vi "AD7609 config.vi"(4 "Timeout for software trig. mode (ms)":u32=15000, 5 "Device serial port":refnum<visa-resource-name>, 6 "Triggering mode":u8(ring) items=["Software", "Hardware, falling edge", "Hardware, rising edge"], 7 "N channels to read":u8(ring)=8 items=["1"=1, "2"=2, "3"=3, "4"=4, "5"=5, "6"=6, "7"=7, "8"=8], 8 "Input voltage range (V)":u8(ring)=1 items=["-5... +5 V", "-10... +10 V"], 9 "Oversampling ratio":u8(ring) items=["1", "2", "4", "8", "16", "32", "64"], 10 "Sampling rate (Hz)":sgl=1000.0, 11 "Number of samples":u32=1000) -> (0 "Config error out":errorcluster, 3 "Config read-back ok":bool=TRUE)   [LabVIEW 2016]
uses:
  <vilib>/Instr/_visa.llb/VISA Open Access Mode.ctl
  AD7609 global.vi
panel:
  out "Configuration read-back":string
  out "Configuration output":string
  # "56 kHz max. 8Ch\n80 kHz max. 1Ch"
  # "PN 25/11/2014, 17/08/2015, 23/08/2016, 03/09/2017"
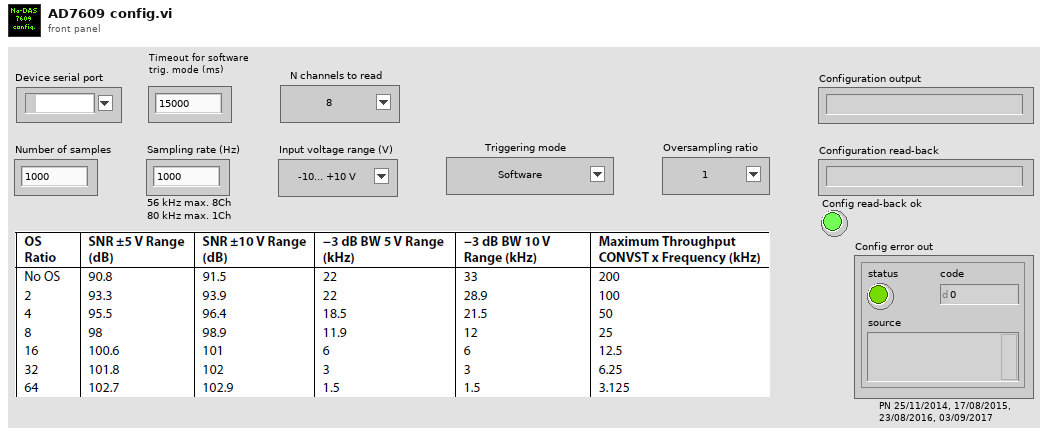
[diagram p1: front panel]
types:
  T1 = typedef "VISA Open Access Mode.ctl" = u32
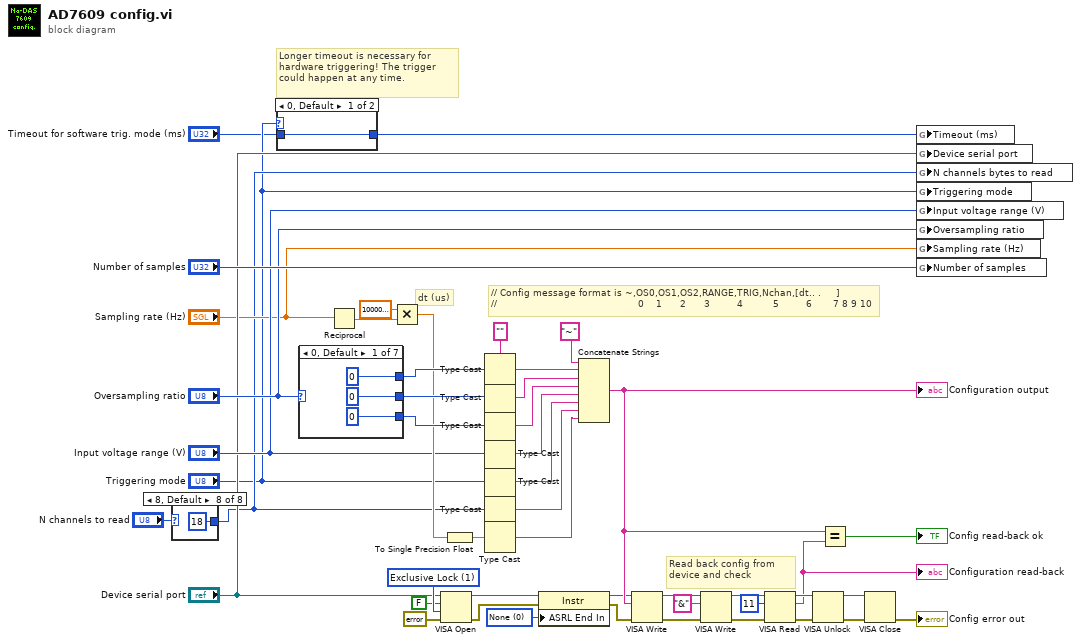
[diagram p0: block diagram]
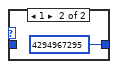
[diagram p2: hidden frame]
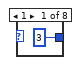
[diagram p3: hidden frame]
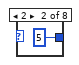
[diagram p4: hidden frame]
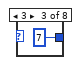
[diagram p5: hidden frame]
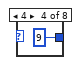
[diagram p6: hidden frame]
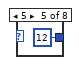
[diagram p7: hidden frame]
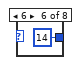
[diagram p8: hidden frame]
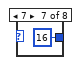
[diagram p9: hidden frame]
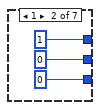
[diagram p10: hidden frame]
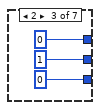
[diagram p11: hidden frame]
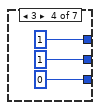
[diagram p12: hidden frame]
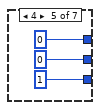
[diagram p13: hidden frame]
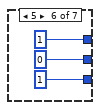
[diagram p14: hidden frame]
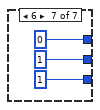
[diagram p15: hidden frame]
diagram:
  w8 = u16 0 items=["None", "Last Bit", "TermChar"] ("Serial Settings:End Mode for Reads")
  w36 = T1 1 items=["VISA Defaults"=0, "Exclusive Lock"=1, "Load Configured Settings"=4] ("Access Mode")
  w12 = ""
  # "Longer timeout is necessary for hardware triggering! The trigger could happen at any time."
  # "Read back config from device and check"
  # "// Config message format is ~,OS0,OS1,OS2,RANGE,TRIG,Nchan,[dt.. .     ]\n//                                               0    1      2      3         4          5         6       7 8 9 10"
  # "dt (us)"
  n1 = case shown="8, Default" "N channels to read" {
    tunnel: [u8 3 u8 5 u8 7 u8 9 u8 12 u8 14 u8 16 u8 18] -> w9
    frame 1 {
    }
    frame 2 {
    }
    frame 3 {
    }
    frame 4 {
    }
    frame 5 {
    }
    frame 6 {
    }
    frame 7 {
    }
    frame 8, Default {
    }
  }
  n2 = case shown="0, Default" "Triggering mode" {
    tunnel: [w57 u32 4294967295 ("Timeout (ms)")] -> w2
    tunnel: "Timeout for software trig. mode (ms)" -> [w57 _]
    frame 0, Default {
    }
    frame 1 {
    }
  }
  n3 = case shown="0, Default" "Oversampling ratio" {
    tunnel: [u8 0 u8 1 u8 0 u8 1 u8 0 u8 1 u8 0] -> w47
    tunnel: [u8 0 u8 0 u8 1 u8 1 u8 0 u8 0 u8 1] -> w46
    tunnel: [u8 0 u8 0 u8 0 u8 0 u8 1 u8 1 u8 1] -> w45
    frame 0, Default {
    }
    frame 1 {
    }
    frame 2 {
    }
    frame 3 {
    }
    frame 4 {
    }
    frame 5 {
    }
    frame 6 {
    }
  }
  n4 = Reciprocal(x="Sampling rate (Hz)") -> (1/x=w39:sgl)
  n5 = Multiply(x=sgl 1000000.0, y=w39) -> (x*y=w37:sgl)
  n6 = VISA Open(duplicate session (F)=FALSE, access mode=w36, error in (no error)=errorcluster {"status"=FALSE, "code"=0, "source"=""}, VISA resource name="Device serial port") -> (VISA resource name=w7:refnum<visa-resource-name>, error out=w4:errorcluster)  [unwired: 1 in]
  n7 = To Single Precision Float(number=w37) -> (single precision float=w25:sgl)
  n8 = Type Cast(type=w12, x=w47) -> (*(type *) &x=w44:string)
  n9 = Type Cast(type=w12, x=w46) -> (*(type *) &x=w43:string)
  n10 = Type Cast(type=w12, x=w45) -> (*(type *) &x=w42:string)
  n11 = Type Cast(type=w12, x="Input voltage range (V)") -> (*(type *) &x=w41:string)
  n12 = Type Cast(type=w12, x="Triggering mode") -> (*(type *) &x=w40:string)
  n13 = Type Cast(type=w12, x=w9) -> (*(type *) &x=w11:string)
  n14 = Type Cast(type=w12, x=w25) -> (*(type *) &x=w13:string)
  n15 = property class="Instr"(reference=w7, error in=w4, "ASRL End In"=w8) -> (reference out=w6:refnum<visa-resource-name>, error out=w5:errorcluster)
  n16 = Concatenate Strings("~", w44, w43, w42, w41, w40, w11, w13) -> (w15:string)
  "Configuration output" <- w15
  n17 = VISA Write(VISA resource name=w6, write buffer=w15, error in (no error)=w5) -> (VISA resource name out=w23:refnum<visa-resource-name>, error out=w24:errorcluster)  [unwired: 1 out]
  n18 = VISA Write(VISA resource name=w23, write buffer="&", error in (no error)=w24) -> (VISA resource name out=w21:refnum<visa-resource-name>, error out=w20:errorcluster)  [unwired: 1 out]
  n19 = VISA Read(VISA resource name=w21, byte count=u32 11, error in (no error)=w20) -> (VISA resource name out=w18:refnum<visa-resource-name>, read buffer=w16:string, error out=w19:errorcluster)  [unwired: 1 out]
  "Configuration read-back" <- w16
  n20 = VISA Unlock(8:w19, 11:w18) -> (0:w33:errorcluster, 3:w34:refnum<visa-resource-name>)
  n21 = Equal?(x=w15, y=w16) -> (x = y?=→"Config read-back ok":bool)
  n22 = VISA Close(VISA resource name=w34, error in (no error)=w33) -> (error out=→"Config error out":errorcluster)
  n23 = global write "AD7609 global.vi" "Timeout (ms)"(w2) -> ()
  n24 = global write "AD7609 global.vi" "Device serial port"("Device serial port") -> ()
  n25 = global write "AD7609 global.vi" "N channels bytes to read"(w9) -> ()
  n26 = global write "AD7609 global.vi" "Triggering mode"("Triggering mode") -> ()
  n27 = global write "AD7609 global.vi" "Input voltage range (V)"("Input voltage range (V)") -> ()
  n28 = global write "AD7609 global.vi" "Oversampling ratio"("Oversampling ratio") -> ()
  n29 = global write "AD7609 global.vi" "Sampling rate (Hz)"("Sampling rate (Hz)") -> ()
  n30 = global write "AD7609 global.vi" "Number of samples"("Number of samples") -> ()
